vi "Calculate Particle Scores Coral.vi"(6 "Limit":dbl=80.0 format="%#_13g", 10 "Sorted Data":dbl[][](array[numeric])) -> (3 "Scores":T1[](array[typedef]))   [LabVIEW 2023]
doc: "Calculate scores based on the particle measurements. Calculated scores are for aspect ratio, area to convex hull area, and moment of inertia. These scores range between 0 and 100 and can be used to categorize particles as targets and non-targets."
uses:
  Target Fields.ctl
  <vilib>/Analysis/baseanly.llb/Mean (DBL).vi
  <vilib>/Analysis/NI_AALBase.lvlib
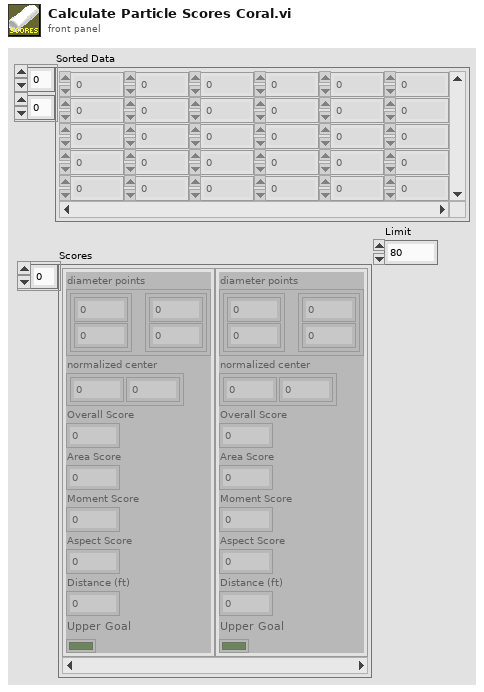
[diagram p1: front panel]
types:
  T1 = typedef "Target Fields.ctl" = cluster{"diameter points":cluster{"first point":cluster{"x":dbl, "y":dbl}, "projected point":cluster{"x":dbl, "y":dbl}}, "normalized center":cluster{"x":dbl, "y":dbl}, "Overall Score":dbl, "Area Score":dbl, "Moment Score":dbl, "Aspect Score":dbl, "Distance (ft)":dbl, "Upper Goal":bool}
  T2 = cluster{cluster{"Numeric":dbl, "Numeric":dbl}, cluster{"Numeric":dbl, "Numeric":dbl}}
  T3 = cluster{cluster{cluster{"Numeric":dbl, "Numeric":dbl}, cluster{"Numeric":dbl, "Numeric":dbl}}, "first point":cluster{"x":dbl, "y":dbl}, "mean":dbl, "Score":dbl, "Score":dbl, "Score":dbl, dbl, bool}
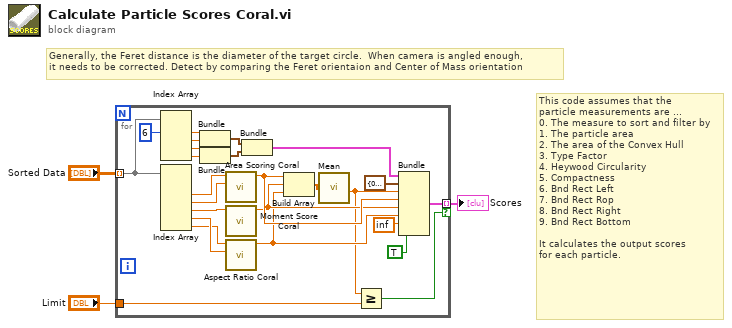
[diagram p0: block diagram]
diagram:
  # "Generally, the Feret distance is the diameter of the target circle.  When camera is angled enough,\nit needs to be corrected. Detect by comparing the Feret orientaion and Center of Mass orientation"
  # "This code assumes that the\nparticle measurements are ...\n0. The measure to sort and filter by\n1. The particle area\n2. The area of the Convex Hull\n3. Type Factor\n4. Heywood Circularity\n5. Compactness\n6. Bnd Rect Left\n7. Bnd Rect Rop\n8. Bnd Rect Right\n9. Bnd Rect Bottom\n\nIt calculates the output scores\nfor each particle."
  n1 = for {
    tunnel: "Sorted Data" -> [w24] mode=indexing
    tunnel: [w23] -> w2 mode=indexing if=w7
    tunnel: "Limit" -> [w12]
    n2 = Index Array(array=w24, index #1=6 ("index")) -> (element #1=w11:dbl, element #2=w10:dbl, element #3=w9:dbl, element #4=w8:dbl)  [unwired: 3 in]
    n3 = Index Array(array=w24) -> (element #2=w20:dbl, element #3=w15:dbl, element #4=w17:dbl, element #5=w14:dbl, element #6=w13:dbl)  [unwired: 6 in, 1 out]
    n4 = Bundle("Numeric"=w11, "Numeric"=w10) -> (w22:cluster{"Numeric":dbl, "Numeric":dbl})  [unwired: 1 in]
    n5 = Bundle("Numeric"=w9, "Numeric"=w8) -> (w21:cluster{"Numeric":dbl, "Numeric":dbl})  [unwired: 1 in]
    n6 = call "Area Scoring Coral.vi"("Convex Hull Area"=w15, "Area"=w20) -> ("Score"=w19:dbl)  [unwired: 9 in]
    n7 = call "Moment Score Coral.vi"("Moment Factor"=w17) -> ("Score"=w18:dbl)  [unwired: 10 in]
    n8 = call "Aspect Ratio Coral.vi"("Circularity"=w14, "Compactness"=w13) -> ("Score"=w16:dbl)  [unwired: 9 in]
    n9 = Bundle(w22, w21) -> (w27:T2)  [unwired: 1 in]
    n10 = Build Array(w19, w18, w16) -> (w5:dbl[])
    n11 = call-poly <vilib>:"Mean.vi"("X"=w5) -> ("mean"=w4:dbl)  [unwired: 1 out]
    n12 = Greater Or Equal?(x=w4, y=w12) -> (x >= y?=w7:bool)
    n13 = Bundle(w27, "first point"=cluster{"x":dbl, "y":dbl} {"x"=0.0, "y"=0.0}, "mean"=w4, "Score"=w19, "Score"=w18, "Score"=w16, inf, TRUE) -> (w23:T3)  [unwired: 1 in]
  }
  "Scores" <- w2
